vi "DIAdem Request Datasheet.vi"(7 "Paths":T1[](array[typedef]), 8 "error in (no error)":errorcluster, 10 "Generator Settings":T4={"Wait? (t)"=TRUE, "ClientPrint? (f)"=FALSE, "Client (\"\")"="", "joinPDF"=FALSE, "Sort Method"=enum."Item", "Export Row (-1=all)"=-1, "Preview"=FALSE, "Estimate Time"=FALSE, "username"="", "jobid"=""}, 11 "Datasheets to Generate":T2[](array[typedef])) -> (0 "error out":errorcluster, 2 "Timed Out?":bool, 3 "Result":string, 5 "Paths":T1[](array[typedef]))   [LabVIEW 2011]
uses:
  Datasheet/Datasheet Generator Settings.ctl
  datasheet script data.ctl
  ITK EXT/utils/keyedarr.llb/Keyed Array.ctl
  Datasheet/Datasheet Report Info.ctl
  DIAdem Daemon Queue.ctl
  DIAdem Daemon Script Type.ctl
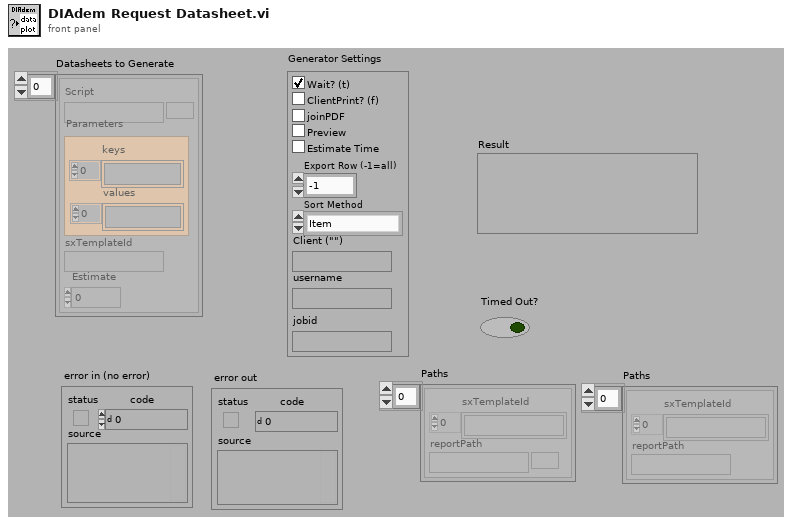
[diagram p1: front panel]
types:
  T1 = typedef "Datasheet Report Info.ctl" = cluster{"sxTemplateId":string[], "reportPath":path}
  T2 = typedef "datasheet script data.ctl" = cluster{"Script":path, "Parameters":T3, "sxTemplateId":string, "Estimate":i32}
  T3 = typedef "Keyed Array.ctl" = cluster{"keys":string[], "values":string[]}
  T4 = typedef "DATASHEET Generator Settings.ctl" = cluster{"Wait? (t)":bool, "ClientPrint? (f)":bool, "Client (\"\")":string, "joinPDF":bool, "Sort Method":enum16{"Item", "Template", "No Sort"}, "Export Row (-1=all)":i32, "Preview":bool, "Estimate Time":bool, "username":string, "jobid":string}
  T5 = typedef "DIAdem Daemon Queue.ctl" = cluster{"Report Template TDM":path, "Report Processor VBS":path, "Report Path PDF":path, "Report Script Params":string, "Username":string, "Script Type":T6, "Report Query Params":string, "Client Machine":string, "Print on Client?":bool, "Response Queue Name":string, "Script Variables":string[], "Start Request Time":timestamp, "Wait?":bool}
  T6 = typedef "DIAdem Daemon Script Type.ctl" = enum16{"Report", "Query", "Script", "Datasheet", "Append", "Restart", "Stop"}
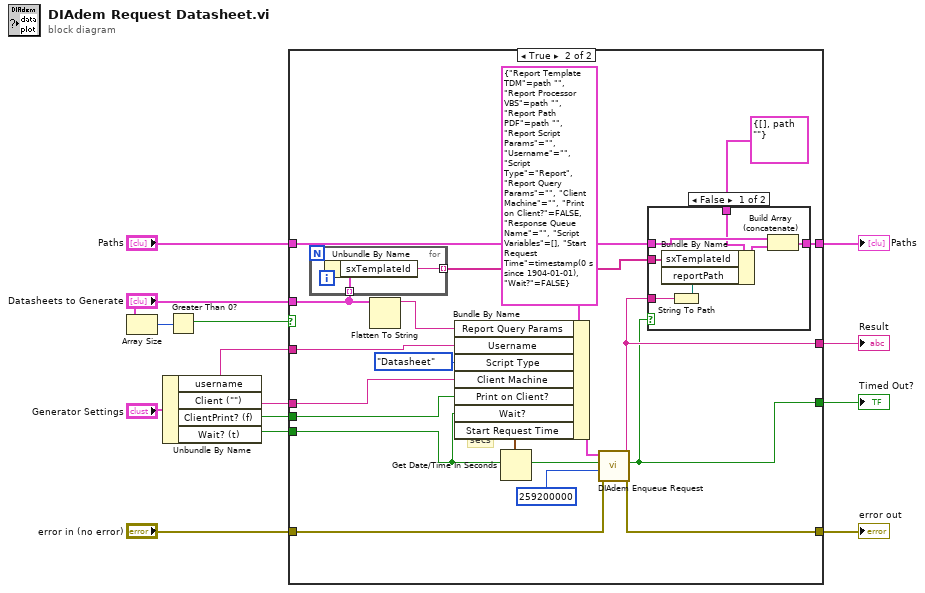
[diagram p0: block diagram]
diagram:
  n1 = Array Size(array="Datasheets to Generate") -> (size(s)=w6:i32)
  n2 = Unbundle By Name("Generator Settings") -> ("username"=w4:string, "Client (\"\")"=w1:string, "ClientPrint? (f)"=w3:bool, "Wait? (t)"=w2:bool)
  n3 = Greater Than 0?(x=w6) -> (x > 0?=w10:bool)
  n4 = case shown="True" w10 {
    tunnel: "error in (no error)" -> [w15 w17]
    tunnel: [w15 w31] -> w13
    tunnel: [_ w26] -> w12
    tunnel: [_ w28] -> w11
    tunnel: "Datasheets to Generate" -> [_ w24]
    tunnel: "Paths" -> [w16 w29]
    tunnel: [w16 w27] -> w7
    tunnel: w4 -> [_ w22]
    tunnel: w3 -> [_ w21]
    tunnel: w2 -> [_ w19]
    tunnel: w1 -> [_ w20]
    frame False {
    }
    frame True {
      # "secs"
      n5 = for {
        tunnel: w24 -> [w37] mode=indexing
        tunnel: [w36] -> w18 mode=indexing
        n6 = Unbundle By Name(w37) -> ("sxTemplateId"=w36:string)
      }
      n7 = Flatten To String(anything=w24) -> (data string=w33:string)  [unwired: 1 in, 4 out]
      n8 = Get Date/Time In Seconds() -> (seconds since 1Jan1904=w30:timestamp)
      n9 = Bundle By Name(cluster=T5 {"Report Template TDM"=path "", "Report Processor VBS"=path "", "Report Path PDF"=path "", "Report Script Params"="", "Username"="", "Script Type"=enum."Report", "Report Query Params"="", "Client Machine"="", "Print on Client?"=FALSE, "Response Queue Name"="", "Script Variables"=[], "Start Request Time"=timestamp(0 s since 1904-01-01), "Wait?"=FALSE} ("DD_Report"), "Report Query Params"=w33, "Username"=w22, "Script Type"=DIAdem_Daemon_Script_Type."Datasheet", "Client Machine"=w20, "Print on Client?"=w21, "Wait?"=w19, "Start Request Time"=w30) -> (w32:T5)
      n10 = call "DIAdem Enqueue Request.vi"("error in (no error)"=w17, "timeout in ms (300000)"=259200000, "Wait for Completion? (f)"=w19, "DD_Report"=w32) -> ("error out"=w31:errorcluster, "timed out?"=w26:bool, "Results"=w28:string)  [unwired: 5 out]
      n11 = case shown="False" w26 {
        tunnel: w29 -> [w44 w45]
        tunnel: w28 -> [w43 _]
        tunnel: [w42 w45] -> w27
        tunnel: T1 {"sxTemplateId"=[], "reportPath"=path ""} ("report") -> [w41 _]
        tunnel: w18 -> [w38 _]
        frame False {
          n12 = String To Path(string=w43) -> (path=w40:path)
          n13 = Bundle By Name(cluster=w41, "sxTemplateId"=w38, "reportPath"=w40) -> (w39:T1)
          n14 = Build Array (concatenate)(w44, w39) -> (w42:T1[])
        }
        frame True {
        }
      }
    }
  }
  "error out" <- w13
  "Timed Out?" <- w12
  "Result" <- w11
  "Paths" <- w7
